vi "CAL-Plot Exemplar.vi"(0 "Test file":path, 5 "Exemplar file":path, 7 "Tolerance (dB)":dbl=5.0, 11 "error in":errorcluster, 12 "Magnitude graph ref":refnum<vi>, 13 "Max SPL?":bool) -> (15 "error out":errorcluster)   [LabVIEW 2015]
uses:
  PXI DAQ VIs/DAQ Engine VIs/PXI Globals.vi
  Utility VIs/Math VIs/Linear to dB (scalar).vi
panel:
  in  "Exemplar Color":u32(colorbox)=13158600
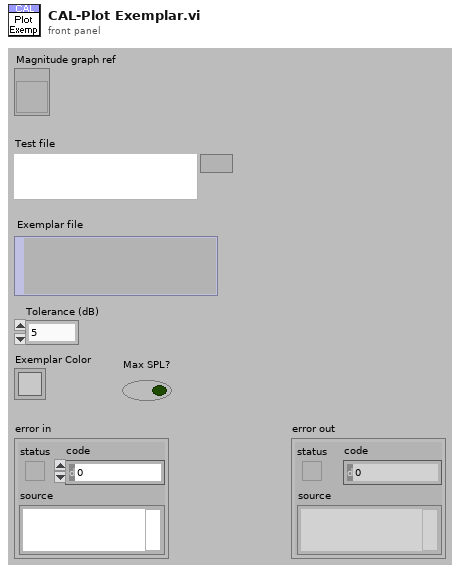
[diagram p1: front panel]
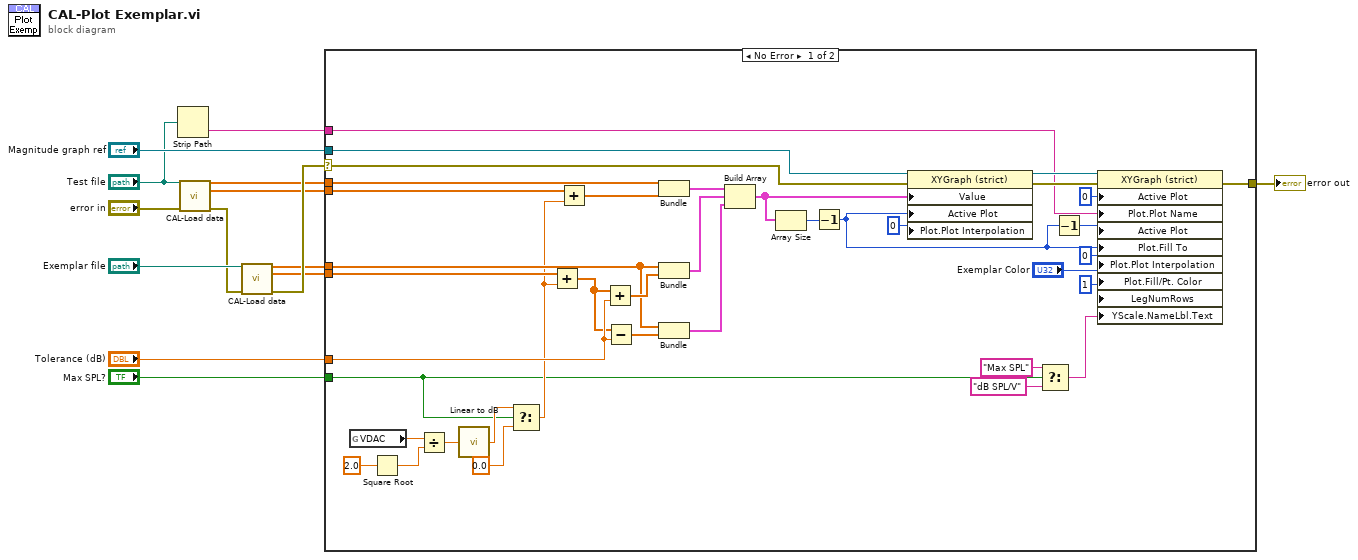
[diagram p0: block diagram]
diagram:
  n1 = Strip Path(path="Test file") -> (name=w1:string)  [unwired: 1 out]
  n2 = call "CAL-Load data.vi"("user path"="Test file", "error in (no error)"="error in") -> ("Frequency (Hz)"=w13:dbl[], "Mag"=w12:dbl[], "error out"=w5:errorcluster)  [unwired: 6 in, 5 out]
  n3 = call "CAL-Load data.vi"("user path"="Exemplar file", "error in (no error)"=w5) -> ("Frequency (Hz)"=w10:dbl[], "Mag"=w9:dbl[], "error out"=w14:errorcluster)  [unwired: 6 in, 5 out]
  n4 = case shown="No Error" w14 {
    selector: w14 -> [w34 w53]
    tunnel: w13 -> [w52 _]
    tunnel: w12 -> [w51 _]
    tunnel: "Tolerance (dB)" -> [w48 _]
    tunnel: w10 -> [w46 _]
    tunnel: w9 -> [w43 _]
    tunnel: "Magnitude graph ref" -> [w35 _]
    tunnel: [w32 w53] -> w4
    tunnel: "Max SPL?" -> [w16 _]
    tunnel: w1 -> [w19 _]
    frame No Error {
      n5 = global read "PXI Globals.vi" "VDAC"() -> (w31:dbl)
      n6 = Square Root(x=2.0) -> (sqrt(x)=w30:dbl)
      n7 = Divide(x=w31, y=w30) -> (x/y=w28:dbl)
      n8 = call-poly "Linear to dB.vi"("Linear"=w28) -> ("dB"=w26:dbl)
      n9 = Select(t=w26, s=w16, f=0.0) -> (s? t:f=w23:dbl)
      n10 = Add(x=w43, y=w23) -> (x+y=w25:dbl[])
      n11 = Add(x=w51, y=w23) -> (x+y=w24:dbl[])
      n12 = Add(x=w25, y=w48) -> (x+y=w47:dbl[])
      n13 = Subtract(x=w25, y=w48) -> (x-y=w45:dbl[])
      n14 = Bundle("Frequency (Hz)"=w52, w24) -> (w50:cluster{"Frequency (Hz)":dbl[], dbl[]})  [unwired: 1 in]
      n15 = Bundle("Frequency (Hz)"=w46, w47) -> (w49:cluster{"Frequency (Hz)":dbl[], dbl[]})  [unwired: 1 in]
      n16 = Bundle("Frequency (Hz)"=w46, w45) -> (w44:cluster{"Frequency (Hz)":dbl[], dbl[]})  [unwired: 1 in]
      n17 = Build Array(w50, w49, w44) -> (w42:cluster{"Frequency (Hz)":dbl[], dbl[]}[])
      n18 = Array Size(array=w42) -> (size(s)=w41:i32)
      n19 = Decrement(x=w41) -> (x-1=w37:i32)
      n20 = property class="XYGraph (strict)"(reference=w35, error in=w34, "Value"=w42, "Active Plot"=w37, "Plot.Plot Interpolation"=u8 0) -> (reference out=w40:refnum<vi>, error out=w33:errorcluster)
      n21 = Select(t="Max SPL", s=w16, f="dB SPL/V") -> (s? t:f=w15:string)
      n22 = Decrement(x=w37) -> (x-1=w21:i32)
      n23 = property class="XYGraph (strict)"(reference=w40, error in=w33, "Active Plot"=u32 0, "Plot.Plot Name"=w19, "Active Plot"=w21, "Plot.Fill To"=w37, "Plot.Plot Interpolation"=u8 0 ("Plot.Point Style"), "Plot.Fill/Pt. Color"="Exemplar Color", "LegNumRows"=u32 1 ("Legend:Number of Rows"), "YScale.NameLbl.Text"=w15) -> (error out=w32:errorcluster)  [unwired: 1 out]
    }
    frame Error {
    }
  }
  "error out" <- w4
